vi "GetType.vi"(0 "reference in":refnum<class "Engine_1DI_2DO.lvclass">) -> (4 "reference out":refnum<class "Engine_1DI_2DO.lvclass">, 6 "obj_type":T1)   [LabVIEW 2019, in "Engine_1DI_2DO.lvclass"]
uses:
  Engine_1DI_2DO.lvclass
  Logger_class/ObjType.ctl
  Logger_class/Logger.lvclass
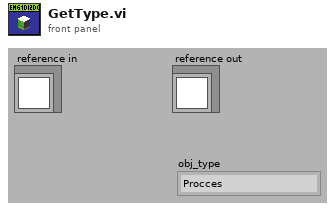
[diagram p1: front panel]
types:
  T1 = typedef "Logger.lvclass/ObjType.ctl" = enum16{"Procces", "Device", "SignalA", "SignalD", "DI", "DO", "DA", "AI", "AO", "AA", "GUI"}
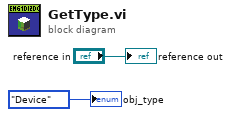
[diagram p0: block diagram]
diagram:
  "reference out" <- "reference in"
  "obj_type" <- ObjType."Device" ("obj_type")
